vi "Set Scroll Bar State.vi"(8 "error in (no error)":errorcluster, 10 "Horizontal Scrollbar Visibility":T1(ring), 11 "Pane in":refnum<vi>) -> (0 "error out":errorcluster, 2 "Pane out":refnum<vi>)   [LabVIEW 2015]
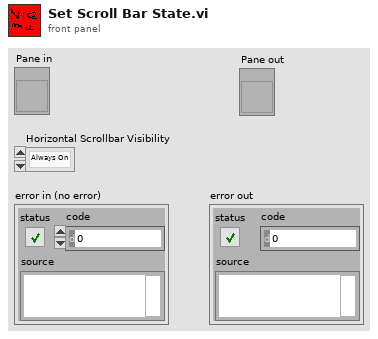
[diagram p1: front panel]
types:
  T1 = enum16{"Always On", "Always Off", "Off While Running"}
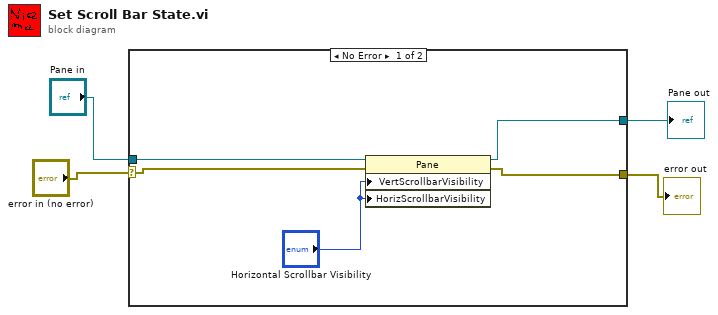
[diagram p0: block diagram]
diagram:
  n1 = case shown="No Error" "error in (no error)" {
    selector: "error in (no error)" -> [w8 w10]
    tunnel: "Pane in" -> [w7 w11]
    tunnel: [w6 w11] -> w2
    tunnel: [w5 w10] -> w1
    frame No Error {
      n2 = property on="Property Node" class="Pane"(reference=w7, error in=w8, "VertScrollbarVisibility"="Horizontal Scrollbar Visibility", "HorizScrollbarVisibility"="Horizontal Scrollbar Visibility") -> (reference out=w6:refnum<vi>, error out=w5:errorcluster)
    }
    frame Error {
    }
  }
  "Pane out" <- w2
  "error out" <- w1
